vi "cRIO FPGA EEPROM Access_Mod8.vi"(6 "Wait (Ticks)":u8=40, 9 "Data in":u8[](array[numeric])=[0, 0, 0, 0], 11 "bytes":u8) -> (1 "Data out":u8[](array[numeric]))   [LabVIEW 2013]
uses:
  <vilib>/eio/EIOMethodNode/EIOMethodNode.xnode
  <vilib>/eio/EIONode/EIONode.xnode
  <vilib>/rvi/eio/common/nirviEmuTemplateMethod_errors.vi
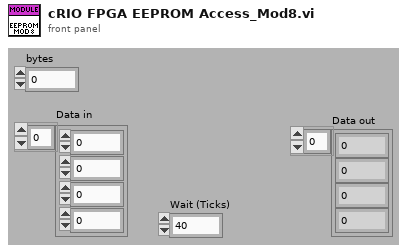
[diagram p1: front panel]
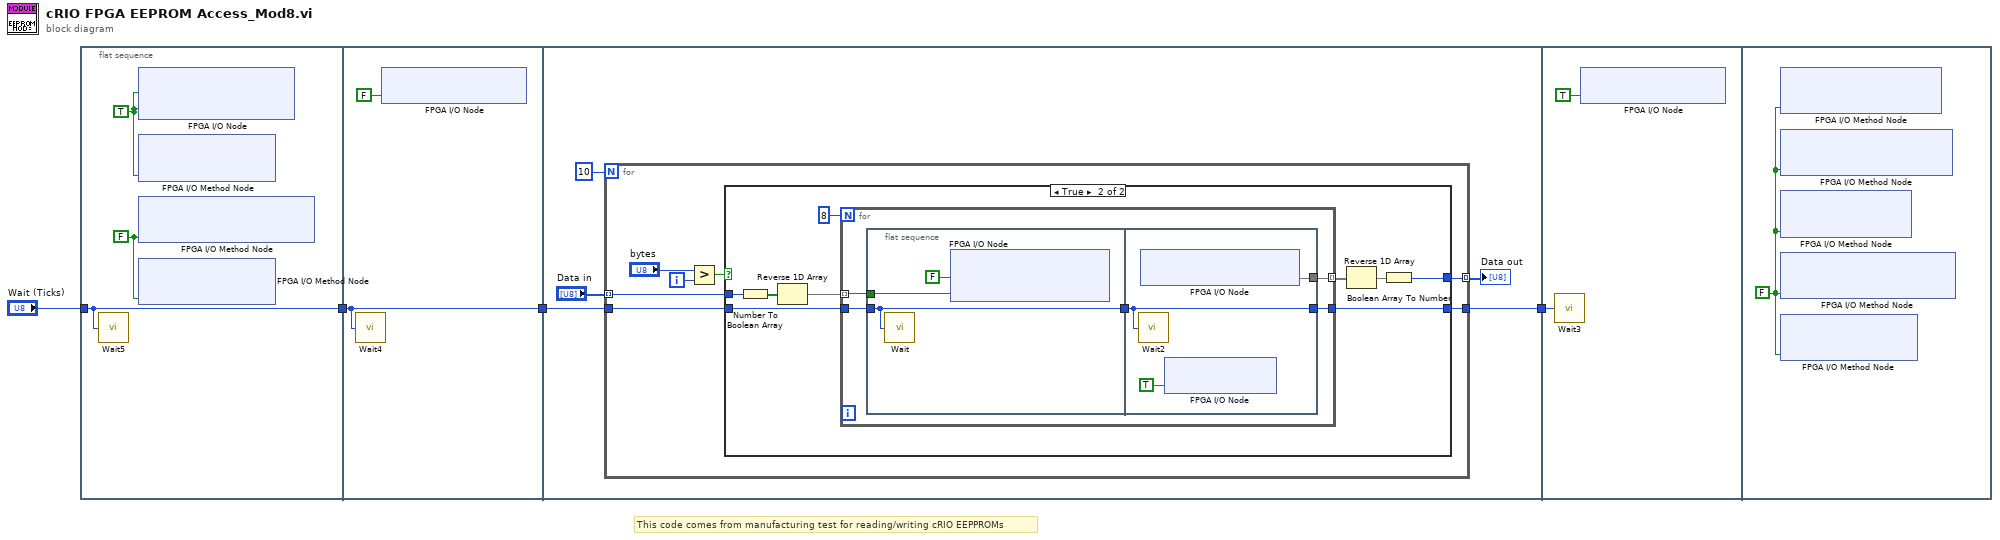
[diagram p0: block diagram]
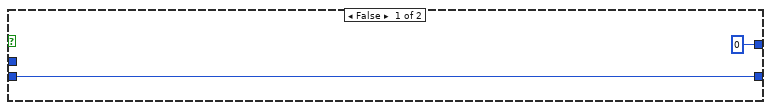
[diagram p2: hidden frame]
diagram:
  # "This code comes from manufacturing test for reading/writing cRIO EEPPROMs"
  n1 = flat-sequence {
    tunnel: "Wait (Ticks)" -> [w5]
    tunnel: [w5] -> w3
    tunnel: w3 -> [w8]
    tunnel: [w8] -> w2
    tunnel: w2 -> [w11]
    tunnel: [w10] -> w1
    tunnel: w1 -> [w44]
    frame #0 {
      w7 = FALSE
      w6 = TRUE ("Digital Out")
      n2 = call "Wait5"("Count(Ticks)"=w5) -> ()  [unwired: 1 out]
      n3 = xnode "FPGA I/O Node"("Mod8/SPI Func (DIO4)"=w6, "Mod8/SPI Clk"=w6) -> ()  [unwired: 2 in, 2 out]
      n4 = xnode "FPGA I/O Method Node"("Enable"=w6) -> ()  [unwired: 1 in, 1 out]
      n5 = xnode "FPGA I/O Method Node"("Enable"=w7) -> ()  [unwired: 1 in, 1 out]
      n6 = xnode "FPGA I/O Method Node"("Data"=w7) -> ()  [unwired: 1 in, 1 out]
    }
    frame #1 {
      n7 = call "Wait4"("Count(Ticks)"=w8) -> ()  [unwired: 1 out]
      n8 = xnode "FPGA I/O Node"("Mod8/SPI CS (DIO5)"=FALSE) -> ()  [unwired: 1 in, 1 out]
    }
    frame #2 {
      n9 = for {
        N: 10 -> [_]
        tunnel: "Data in" -> [w21] mode=indexing
        tunnel: [w20] -> w13 mode=indexing
        tunnel: w11 -> [w16]
        tunnel: [w15] -> w10
        i -> [w18]
        n10 = Greater?(x="bytes", y=w18) -> (0:w17:bool)
        n11 = case shown="True" w17 {
          tunnel: w21 -> [_ w31]
          tunnel: [u8 0 w30] -> w20
          tunnel: w16 -> [w22 w25]
          tunnel: [w22 w24] -> w15
          frame False {
          }
          frame True {
            n12 = Number To Boolean Array(number=w31) -> (Boolean array=w29:bool[])
            n13 = Reverse 1D Array(array=w29) -> (reversed array=w28:bool[])
            n14 = for {
              N: 8 -> [_]
              tunnel: [w37] -> w27 mode=indexing
              tunnel: w28 -> [w36] mode=indexing
              tunnel: w25 -> [w35]
              tunnel: [w33] -> w24
              n15 = flat-sequence {
                tunnel: w36 -> [w39]
                tunnel: w35 -> [w38]
                tunnel: [w38] -> w34
                tunnel: [w42] -> w37
                tunnel: w34 -> [w41]
                tunnel: [w41] -> w33
                frame #0 {
                  n16 = call "Wait"("Count(Ticks)"=w38) -> ()  [unwired: 1 out]
                  n17 = xnode "FPGA I/O Node"("Mod8/SPI Clk"=FALSE ("Digital Out"), "Mod8/SPI MOSI (DIO7)"=w39) -> ()  [unwired: 2 in, 2 out]
                }
                frame #1 {
                  n18 = call "Wait2"("Count(Ticks)"=w41) -> ()  [unwired: 1 out]
                  n19 = xnode "FPGA I/O Node"() -> ("Mod8/SPI MISO (DIO6)"=w42)  [unwired: 1 in, 1 out]
                  n20 = xnode "FPGA I/O Node"("Mod8/SPI Clk"=TRUE ("Digital Out")) -> ()  [unwired: 1 in, 1 out]
                }
              }
            }
            n21 = Reverse 1D Array(array=w27) -> (reversed array=w26:void[])
            n22 = Boolean Array To Number(Boolean array=w26) -> (number=w30:u8)
          }
        }
      }
      "Data out" <- w13
    }
    frame #3 {
      n23 = call "Wait3"("Count(Ticks)"=w44) -> ()  [unwired: 1 out]
      n24 = xnode "FPGA I/O Node"("Mod8/SPI CS (DIO5)"=TRUE ("Digital Out")) -> ()  [unwired: 1 in, 1 out]
    }
    frame #4 {
      w46 = FALSE ("Digital Enable")
      n25 = xnode "FPGA I/O Method Node"("Enable"=w46) -> ()  [unwired: 1 in, 1 out]
      n26 = xnode "FPGA I/O Method Node"("Enable"=w46) -> ()  [unwired: 1 in, 1 out]
      n27 = xnode "FPGA I/O Method Node"("Enable"=w46) -> ()  [unwired: 1 in, 1 out]
      n28 = xnode "FPGA I/O Method Node"("Enable"=w46) -> ()  [unwired: 1 in, 1 out]
      n29 = xnode "FPGA I/O Method Node"("Enable"=w46) -> ()  [unwired: 1 in, 1 out]
    }
  }
